vi "buildVersion.vi"() -> (3 "build":string)   [LabVIEW 2018]
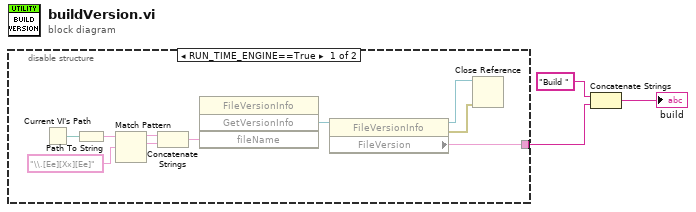
[diagram p0: block diagram]
diagram:
  n1 = disable-structure shown="RUN_TIME_ENGINE==True" {
    disable-tunnel: [w6 _] -> w2
    frame condition #0 {
      n2 = Current VI's Path() -> (path=w9:path)
      n3 = Path To String(path=w9) -> (string=w13:string)
      n4 = Match Pattern(string=w13, regular expression="\\.[Ee][Xx][Ee]") -> (before substring=w11:string, match substring=w10:string)  [unwired: 1 in, 2 out]
      n5 = Concatenate Strings(w11, w10) -> (w12:string)
      n6 = invoke class="FileVersionInfo" method="GetVersionInfo"("fileName"=w12) -> ("GetVersionInfo"=w8:refnum<k24>)  [unwired: 3 in, 3 out]
      n7 = property class="FileVersionInfo"(reference=w8) -> (reference out=w5:refnum<k24>, error out=w4:errorcluster, "FileVersion"=w6:string)  [unwired: 1 in]
      n8 = Close Reference(reference=w5, error in (no error)=w4) -> ()  [unwired: 1 out]
    }
    frame condition #1 (active) {
    }
  }
  n9 = Concatenate Strings("Build " ("build"), w2) -> (→"build":string)
